vi "Register.vi"(8 "error in (no error)":errorcluster, 9 "ConnectionString":string, 10 "Service":T1, 11 "MicronCLI in":refnum<class "MicronCLI.lvclass">) -> (0 "error out":errorcluster, 3 "MicronCLI out":refnum<class "MicronCLI.lvclass">)   [LabVIEW 2019, in "MicronCLI.lvclass"]
uses:
  MicronCLI.lvclass
  Typedefs/ServiceDetails.ctl
  MicronCLI.lvclass/MicronCLI.ctl
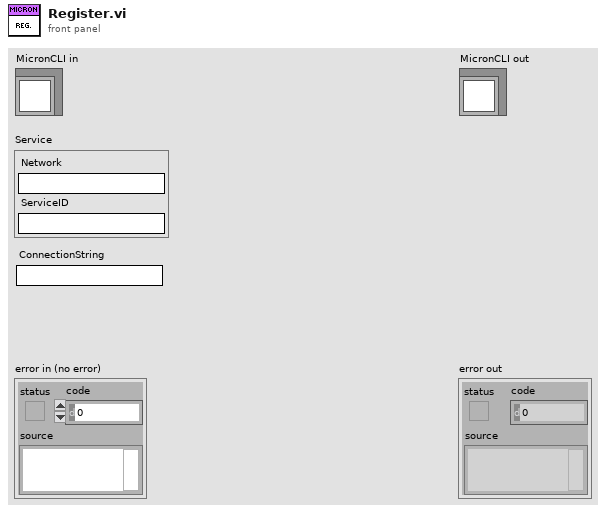
[diagram p1: front panel]
types:
  T1 = typedef "MicronCLI.lvclass/ServiceDetails.ctl" = cluster{"Network":string, "ServiceID":string}
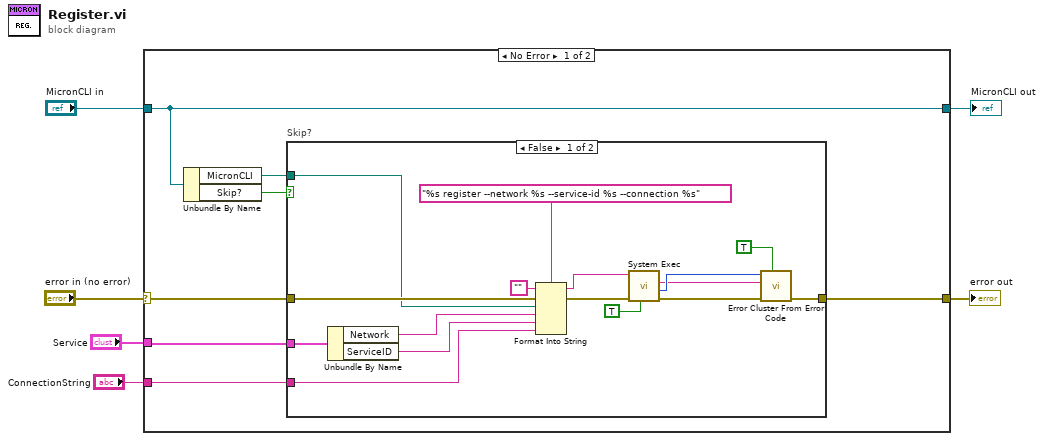
[diagram p0: block diagram]
diagram:
  n1 = case shown="No Error" "error in (no error)" {
    selector: "error in (no error)" -> [w13 w32]
    tunnel: [w9 w32] -> w5
    tunnel: [w12 w31] -> w3
    tunnel: "MicronCLI in" -> [w12 w31]
    tunnel: "Service" -> [w10 _]
    tunnel: "ConnectionString" -> [w7 _]
    frame No Error {
      n2 = Unbundle By Name(w12) -> ("MicronCLI"=w11:path, "Skip?"=w8:bool)
      n3 = case "Skip?" shown="False" w8 {
        tunnel: w13 -> [w29 w30]
        tunnel: w11 -> [w25 _]
        tunnel: w10 -> [w23 _]
        tunnel: [w18 w30] -> w9
        tunnel: w7 -> [w14 _]
        frame False {
          n4 = Unbundle By Name(w23) -> ("Network"=w22:string, "ServiceID"=w21:string)
          n5 = Format Into String(format string="%s register --network %s --service-id %s --connection %s", initial string="", error in=w29, w25, w22, w21, w14) -> (resulting string=w20:string, error out=w27:errorcluster)
          n6 = call <vilib>:"System Exec.vi"("run minimized? (F)"=TRUE, "error in (no error)"=w27, "command line"=w20) -> ("error out"=w28:errorcluster, "return code"=w17:i32, "standard error"=w16:string)  [unwired: 5 in, 1 out]
          n7 = call <vilib>:"Error Cluster From Error Code.vi"("show call chain? (False)"=TRUE, "error in (no error)"=w28, "error message (\"\")"=w16, "error code (0)"=w17) -> ("error out"=w18:errorcluster)  [unwired: 5 in]
        }
        frame True {
        }
      }
    }
    frame Error {
    }
  }
  "error out" <- w5
  "MicronCLI out" <- w3
